vi "Get Cursor Position.vi"(8 "error in (no error)":errorcluster, 10 "Cursor":T1, 11 "DPO4104 in":refnum<class "DPO4104.lvclass">) -> (0 "error out":errorcluster, 2 "Position":dbl format="%.9f", 3 "DPO4104 out":refnum<class "DPO4104.lvclass">)   [LabVIEW 2018, in "DPO4104.lvlib" / "DPO4104.lvclass"]
doc: "This Override method is used to get cursor(s) position from the Oscope instrument. Use 'Cursor' control to select the cursor of interest, and carry out its value to the 'Position' indicator."
uses:
  DPO4104.lvclass
  PPLs/Oscilloscope/Parent/Oscilloscope.lvlibp/Custom Controls/Select Cursor.ctl
  PPLs/Oscilloscope/Parent/Oscilloscope.lvlibp/Oscilloscope.lvclass
  C:/Projects/LabVIEW/PPLs/Oscilloscope/Parent/Oscilloscope.lvlibp/Oscilloscope.lvclass
  PPLs/Oscilloscope/Parent/Oscilloscope.lvlibp
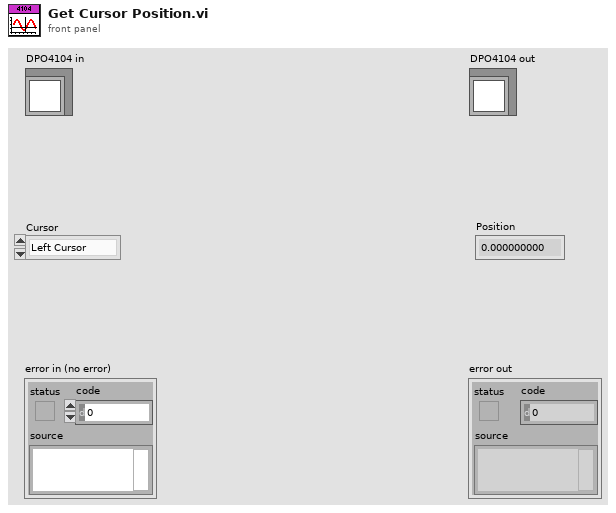
[diagram p1: front panel]
types:
  T1 = typedef "Oscilloscope.lvlibp/Select Cursor.ctl" = enum16{"Left Cursor", "Right Cursor", "Top Cursor", "Bottom Cursor"}
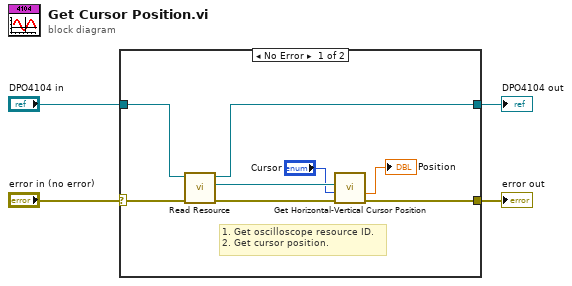
[diagram p0: block diagram]
diagram:
  n1 = case shown="No Error" "error in (no error)" {
    selector: "error in (no error)" -> [w11 w13]
    tunnel: [w7 w13] -> w3
    tunnel: "DPO4104 in" -> [w12 w14]
    tunnel: [w10 w14] -> w1
    frame No Error {
      # "1. Get oscilloscope resource ID.\n2. Get cursor position."
      n2 = call "Read Resource.vi"("error in (no error)"=w11, "Oscilloscope in"=w12) -> ("error out"=w8:errorcluster, "Resource"=w9:refnum<visa-resource-name>, "Oscilloscope out"=w10:refnum<class "DPO4104.lvclass">)  [unwired: 7 in]
      n3 = call "Get Horizontal-Vertical Cursor Position.vi"("error in (no error)"=w8, "Cursor"="Cursor", "VISA resource name"=w9) -> ("error out"=w7:errorcluster, "Position"=→"Position":dbl)  [unwired: 6 in, 1 out]
    }
    frame Error {
    }
  }
  "error out" <- w3
  "DPO4104 out" <- w1
